vi "Multiply - R,RM.vi"(1 "Real Matrix A":T1, 2 "Real Scalar c":dbl) -> (0 "c * A":T1)   [LabVIEW 2010, in "NI_Matrix.lvlib"]
doc: "Returns the product of the inputs."
uses:
  NI_Matrix.lvlib
  RealMatrix.ctl
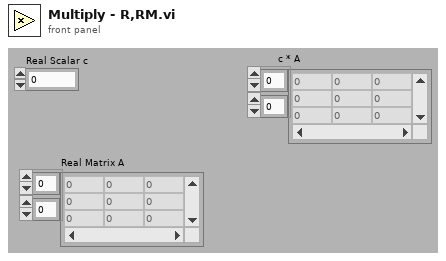
[diagram p1: front panel]
types:
  T1 = typedef "NI_Matrix.lvlib/RealMatrix.ctl" = dbl[][]
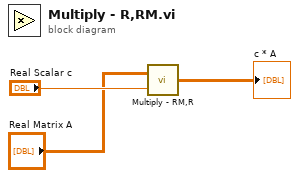
[diagram p0: block diagram]
diagram:
  n1 = call "Multiply - RM,R.vi"("Real Scalar c"="Real Scalar c", "Real Matrix A"="Real Matrix A") -> ("A * c"=→"c * A":T1)
